vi "Configure Trigger Core.vi"(8 "error in (no error)":errorcluster, 9 "trigger holdoff (500.0 E-9 s)":dbl[unit]=5e-07 format="%^.2e", 10 "trigger type (Edge)":i32(ring)=1 items=["Edge"=1, "TV"=5, "Runt"=3, "Glitch"=4, "Width"=2, "AC Line"=7, "Immediate"=6], 11 "CS++Scope":refnum<class "CS++Scope.lvclass">) -> (0 "error out":errorcluster, 3 "CS++Scope out":refnum<class "CS++Scope.lvclass">)   [LabVIEW 2014, in "CS++Scope.lvlib" / "CS++Scope.lvclass"]
doc: "This VI configures the common properties of the trigger subsystem. These properties are the trigger type and holdoff.\nWhen you call IviScope Read Waveform, IviScope Read Waveform Measurement [WM], IviScope Read Min Max Waveform [MmW], or IviScope Initiate Acquisition, the oscilloscope waits for a trigger. You specify the type of trigger for which the oscilloscope waits with the Trigger Type parameter.\nIf the oscilloscope requires multiple waveform acquisitions to build a complete waveform, it waits for the length of time you specify with the Holdoff parameter to elapse since the previous trigger. The oscilloscope then waits for the next trigger. Once the oscilloscope acquires a complete waveform, it returns to the Idle state."
uses:
  CS++Scope.lvclass
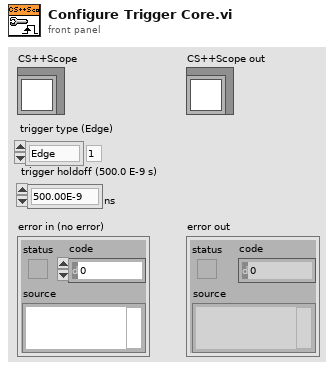
[diagram p1: front panel]
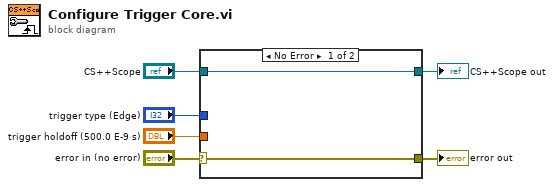
[diagram p0: block diagram]
diagram:
  n1 = case shown="No Error" "error in (no error)" {
    selector: "error in (no error)" -> [w7 w10]
    tunnel: [w7 w10] -> w5
    tunnel: [w8 w9] -> w2
    tunnel: "CS++Scope" -> [w8 w9]
    tunnel: "trigger type (Edge)" -> [_ _]
    tunnel: "trigger holdoff (500.0 E-9 s)" -> [_ _]
    frame No Error {
    }
    frame Error {
    }
  }
  "error out" <- w5
  "CS++Scope out" <- w2
